vi "Weighted_Cross_Moments simple.vi"(0 "AI Cluster 1":T3={"Colour"=0, "Inst type"=enum."Pitot-static tube", "Inst name"="Manometer voltage", "Symbol"="U", "Code name"="", "Extra Info"="U", "Inst Array"=enum."PWA", "Extra Titles"=[], "Extra Values"=[], "U"=0.0, "u^2"=0.0, "u^3"=0.0, "u^4"=0.0, "Skew_u"=0.0, "Kurt_u"=0.0, "Sd Error in Mean"=0.0, "% u'/U"=0.0, "X"=0.0, "Y"=0.0, "Z"=0.0, "Timescale integral Estimate"=0.0, "Sd Error in Variance"=0.0, "Calib File"=path "", "Calib Constants"=[], "Output Position"=FALSE, "Stats"=enum."None", "Av Sampling Rate"=0.0, "Av No of Samples"=0.0, "Total Meas Time (s)"=0.0, "ADAM Ch Name"="", "Max value"=0.0, "Min value"=0.0, "Req Sample Rate Hz"=0.0, "Sync Delay Time (s)"=0.0, "Ch No"=0, "Device"="", "Use Latest Calib"=FALSE, "Port"="", "Metadata Ch Names"=[], "Metadata Ch Values"=[], "Label"=""} {"Sync Delay Time (s)" format="%.4f"; "Total Meas Time (s)" format="%_5g"; "Sd Error in Variance" format="%_3g"; "Skew_u" format="%_3g"; "% u'/U" format="%_3g"; "Sd Error in Mean" format="%_3g"; "Kurt_u" format="%_3g"; "u^4" format="%_3g"; "u^3" format="%_3g"; "U" format="%_3g"; "u^2" format="%_3g"}, 1 "AI Cluster 2":T3={"Colour"=0, "Inst type"=enum."Pitot-static tube", "Inst name"="Manometer voltage", "Symbol"="U", "Code name"="", "Extra Info"="U", "Inst Array"=enum."PWA", "Extra Titles"=[], "Extra Values"=[], "U"=0.0, "u^2"=0.0, "u^3"=0.0, "u^4"=0.0, "Skew_u"=0.0, "Kurt_u"=0.0, "Sd Error in Mean"=0.0, "% u'/U"=0.0, "X"=0.0, "Y"=0.0, "Z"=0.0, "Timescale integral Estimate"=0.0, "Sd Error in Variance"=0.0, "Calib File"=path "", "Calib Constants"=[], "Output Position"=FALSE, "Stats"=enum."None", "Av Sampling Rate"=0.0, "Av No of Samples"=0.0, "Total Meas Time (s)"=0.0, "ADAM Ch Name"="", "Max value"=0.0, "Min value"=0.0, "Req Sample Rate Hz"=0.0, "Sync Delay Time (s)"=0.0, "Ch No"=0, "Device"="", "Use Latest Calib"=FALSE, "Port"="", "Metadata Ch Names"=[], "Metadata Ch Values"=[], "Label"=""} {"Sync Delay Time (s)" format="%.4f"; "Total Meas Time (s)" format="%_5g"; "Sd Error in Variance" format="%_3g"; "Skew_u" format="%_3g"; "% u'/U" format="%_3g"; "Sd Error in Mean" format="%_3g"; "Kurt_u" format="%_3g"; "u^4" format="%_3g"; "u^3" format="%_3g"; "U" format="%_3g"; "u^2" format="%_3g"}, 2 "Time Cluster 1":T1, 3 "Time Cluster 2":T1, 5 "Shift Cluster In":cluster{"Stats":dbl[]} {"Stats" format="%.2f"}, 7 "Array 2 Time (s) offset (Default 0)":dbl, 9 "interp. method":enum16{"nearest", "linear"}(ring)=enum."linear", 11 "Index1":i32, 13 "Index2":i32) -> (17 "output cluster":T2 {"Time Window (ms)" format="%.2f"; "w^2 Paired" format="%.2f"; "u^2 Paired" format="%.2f"; "u^2w^2" format="%.2f"; "u^3w" format="%.2f"; "uw^3" format="%.2f"; "uw/u'w'" format="%.2f"; "uw^2" format="%.2f"; "u^2w" format="%.2f"; "uw" format="%.2f"}, 19 "Shift Cluster Out":cluster{"Stats":dbl[]} {"Stats" format="%.2f"})   [LabVIEW 2021]
uses:
  Controls/Analysis_info_cluster.ctl
  Controls/Inst_type.ctl
  Controls/Instrument_Array.ctl
  Controls/Correlation_cluster1.ctl
  Controls/Time_Trace_Cluster.ctl
  Globals/Meas_global.vi
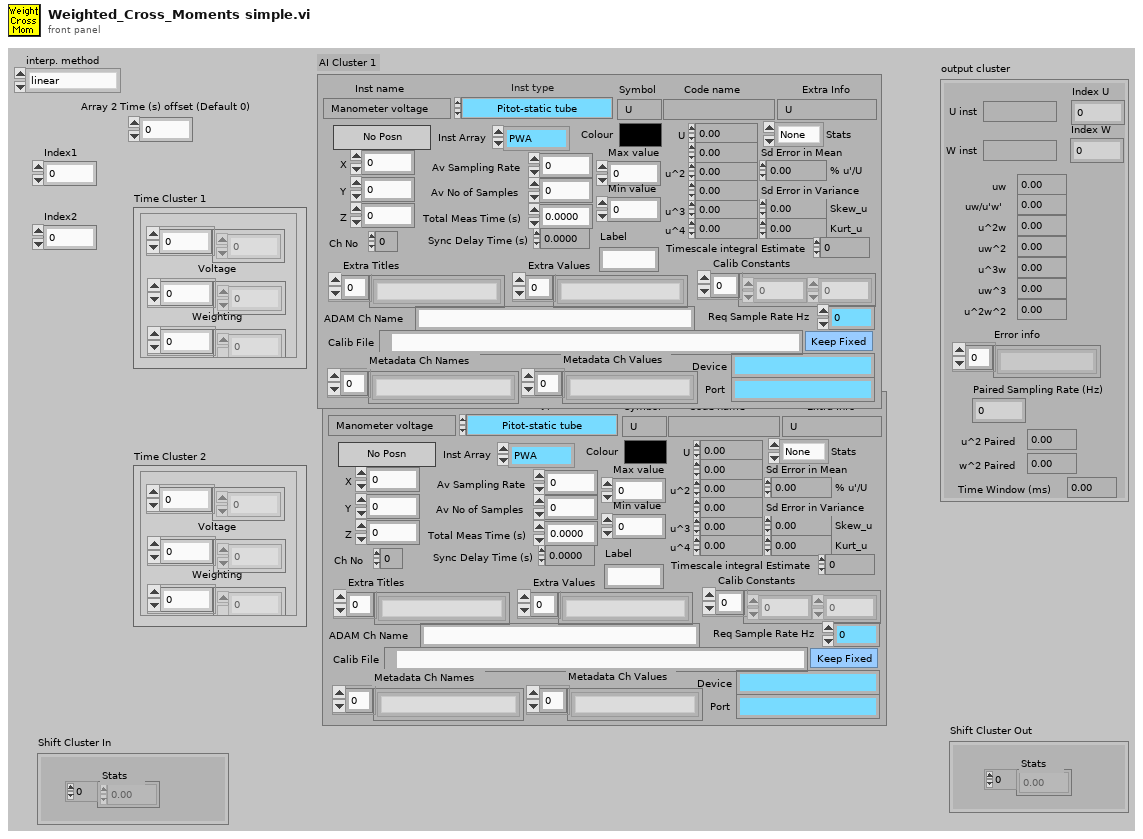
[diagram p1: front panel]
types:
  T1 = typedef "Time_Trace_Cluster.ctl" = cluster{"Weighting":dbl[], "Voltage":dbl[], "Eng Values":dbl[]}
  T2 = typedef "Correlation_cluster1.ctl" = cluster{"U inst":string, "uw":dbl, "u^2w":dbl, "uw^2":dbl, "uw/u'w'":dbl, "W inst":string, "uw^3":dbl, "u^3w":dbl, "u^2w^2":dbl, "Index U":i32, "Index W":i32, "Error info":string[], "Paired Sampling Rate (Hz)":dbl, "u^2 Paired":dbl, "w^2 Paired":dbl, "Time Window (ms)":dbl}
  T3 = typedef "Analysis_info_cluster.ctl" = cluster{"Colour":u32, "Inst type":T4, "Inst name":string, "Symbol":string, "Code name":string, "Extra Info":string, "Inst Array":T5, "Extra Titles":string[], "Extra Values":string[], "U":dbl, "u^2":dbl, "u^3":dbl, "u^4":dbl, "Skew_u":dbl, "Kurt_u":dbl, "Sd Error in Mean":dbl, "% u'/U":dbl, "X":dbl, "Y":dbl, "Z":dbl, "Timescale integral Estimate":dbl, "Sd Error in Variance":dbl, "Calib File":path, "Calib Constants":dbl[], "Output Position":bool, "Stats":enum16{"None", "Basic", "Full"}, "Av Sampling Rate":dbl, "Av No of Samples":dbl, "Total Meas Time (s)":dbl, "ADAM Ch Name":string, "Max value":dbl, "Min value":dbl, "Req Sample Rate Hz":dbl, "Sync Delay Time (s)":dbl, "Ch No":i16, "Device":string, "Use Latest Calib":bool, "Port":string, "Metadata Ch Names":string[], "Metadata Ch Values":string[], "Label":string}
  T4 = typedef "Inst_type.ctl" = enum16{"Raw voltage", "Raw with zero offsetting", "Propeller anemometer", "Pressure Transducer", "Pitot-static tube", "Hot wire", "Cross wire 1", "Cross wire 2", "Generic Linear", "Generic Polynomial", "Generic BackPoly", "Fast FID", "Thermocouple", "Cold wire", "Pulsed Wire", "LDA Vel", "LDA Tran time", "LDA Arr time", "Microphone"}
  T5 = typedef "Instrument_Array.ctl" = enum16{"PWA", "LDA", "Analogue"}
  T6 = typedef "Resample mode.ctl" = cluster{"Mode":enum16{"Index", "Interpolate"}, "Index":dbl[]}
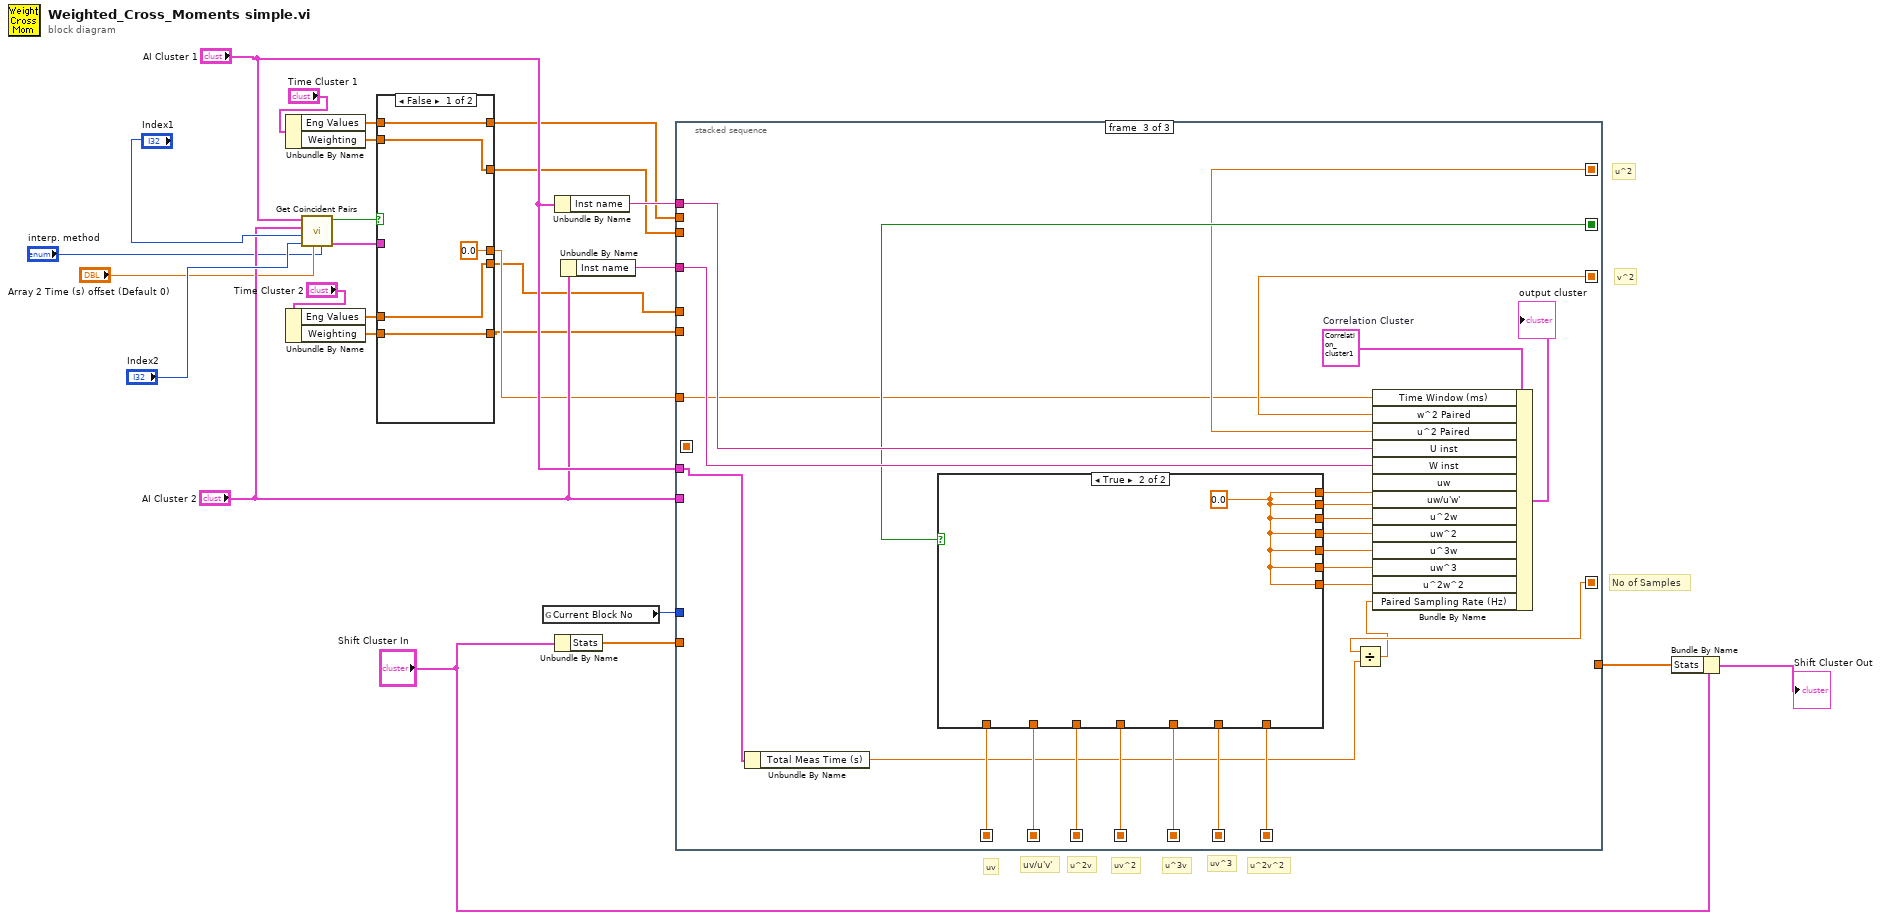
[diagram p0: block diagram]
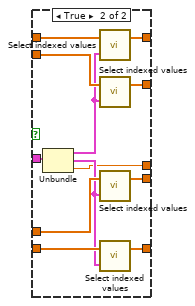
[diagram p2: hidden frame]
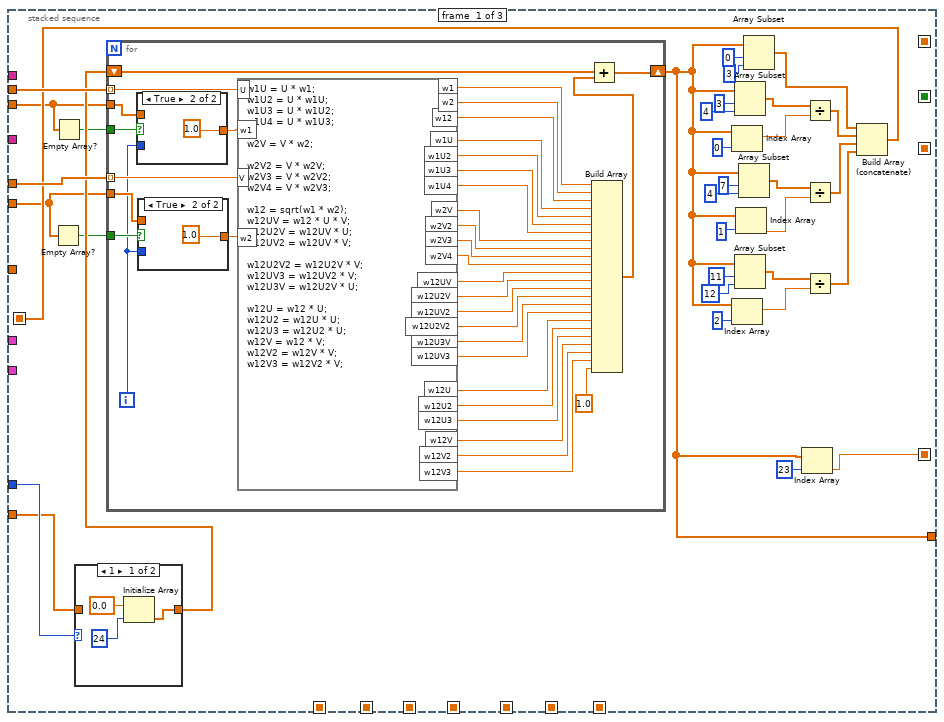
[diagram p3: hidden frame]
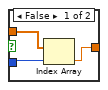
[diagram p5: hidden frame]
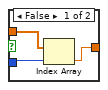
[diagram p6: hidden frame]
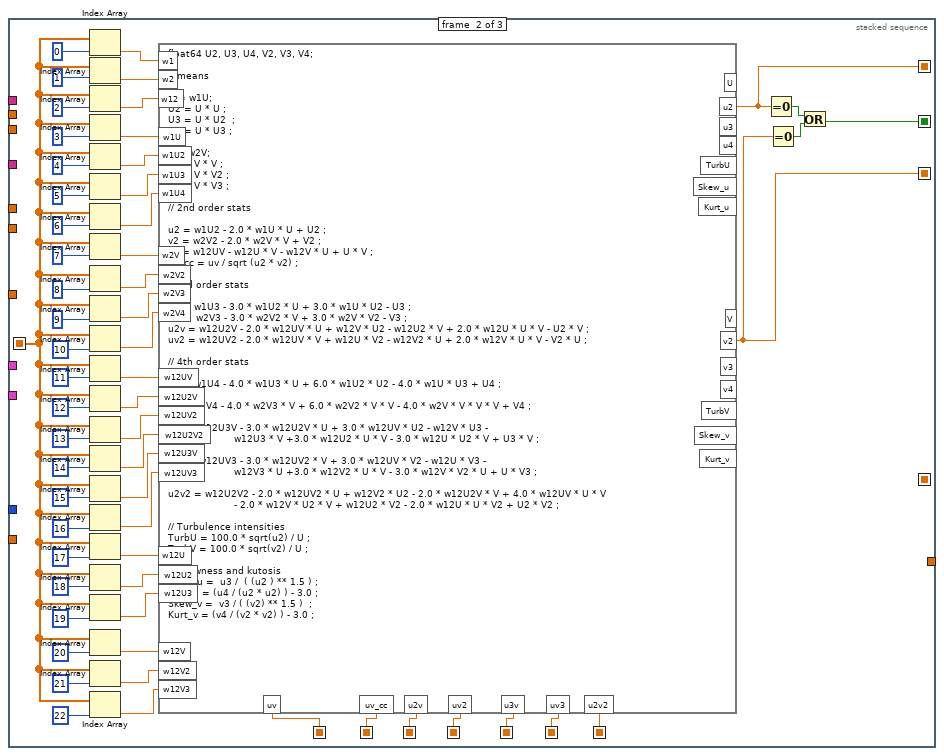
[diagram p7: hidden frame]
diagram:
  # "v^2"
  # "u^2"
  # "No of Samples"
  # "u^2v^2"
  # "uv^3"
  # "u^3v"
  # "uv^2"
  # "u^2v"
  # "uv/u'v'"
  # "uv"
  n1 = Unbundle By Name("Time Cluster 1") -> ("Eng Values"=w16:dbl[], "Weighting"=w17:dbl[])
  n2 = Unbundle By Name("Time Cluster 2") -> ("Eng Values"=w18:dbl[], "Weighting"=w19:dbl[])
  n3 = call "Get Coincident Pairs.vi"("interp. method"="interp. method", "Array 2 Time (s) offset (Default 0)"="Array 2 Time (s) offset (Default 0)", "Index2"="Index2", "Index1"="Index1", "Cluster 2"="AI Cluster 2", "Cluster 1"="AI Cluster 1") -> ("Pairs"=w14:cluster{"Cluster":T6, "Cluster":T6, dbl}, "Need to Update"=w15:bool)  [unwired: 4 in]
  n4 = case shown="False" w15 {
    tunnel: w14 -> [_ w43]
    tunnel: w16 -> [w31 w42]
    tunnel: w17 -> [w30 w41]
    tunnel: w18 -> [w29 w40]
    tunnel: w19 -> [w28 w39]
    tunnel: [w31 w35] -> w3
    tunnel: [w30 w36] -> w8
    tunnel: [w29 w37] -> w2
    tunnel: [w28 w38] -> w5
    tunnel: [0.0 w32] -> w6
    frame False {
    }
    frame True {
      n5 = Unbundle(w43) -> ("Cluster"=w33:T6, "Cluster"=w34:T6, w32:dbl)
      n6 = call "Select indexed values.vi"("Cluster"=w33, "Values"=w42) -> ("Values Out"=w35:dbl[])  [unwired: 1 in]
      n7 = call "Select indexed values.vi"("Cluster"=w33, "Values"=w41) -> ("Values Out"=w36:dbl[])  [unwired: 1 in]
      n8 = call "Select indexed values.vi"("Cluster"=w34, "Values"=w40) -> ("Values Out"=w37:dbl[])  [unwired: 1 in]
      n9 = call "Select indexed values.vi"("Cluster"=w34, "Values"=w39) -> ("Values Out"=w38:dbl[])  [unwired: 1 in]
    }
  }
  n10 = global read "Meas_global.vi" "Current Block No"() -> (w24:i32)
  n11 = Unbundle By Name("AI Cluster 1") -> ("Inst name"=w26:string)
  n12 = Unbundle By Name("Shift Cluster In") -> ("Stats"=w21:dbl[])
  n13 = Unbundle By Name("AI Cluster 2") -> ("Inst name"=w25:string)
  n14 = stacked-sequence {
    seq-local: [_ w172 _] -> [_ _ w205]
    seq-local: [_ w171 _] -> [_ _ w204]
    seq-local: [w73 _ _] -> [_ w133 _]
    seq-local: [_ w166 _] -> [_ _ w201]
    seq-local: [_ w165 _] -> [_ _ w200]
    seq-local: [_ w146 _] -> [_ _ w198]
    seq-local: [_ w145 _] -> [_ _ w196]
    seq-local: [_ w144 _] -> [_ _ w194]
    seq-local: [_ w128 _] -> [_ _ w192]
    seq-local: [w48 _ _] -> [_ _ w190]
    seq-local: [_ w127 _] -> [_ _ w187]
    seq-local: [_ w126 _] -> [_ _ w186]
    tunnel: w3 -> [w77 _ _]
    tunnel: w2 -> [w76 _ _]
    tunnel: w24 -> [w75 _ _]
    tunnel: w8 -> [w47 _ _]
    tunnel: w5 -> [w46 _ _]
    tunnel: w26 -> [_ _ w209]
    tunnel: w25 -> [_ _ w208]
    tunnel: "AI Cluster 1" -> [_ _ w191]
    tunnel: "AI Cluster 2" -> [_ _ _]
    tunnel: w21 -> [w51 _ _]
    tunnel: [w49 _ _] -> w20
    tunnel: w6 -> [_ _ w185]
    frame #0 {
      n15 = Empty Array?(array=w46) -> (empty?=w44:bool)
      n16 = Empty Array?(array=w47) -> (empty?=w45:bool)
      n17 = case shown="1" w75 {
        tunnel: [w79 w81] -> w74
        tunnel: w51 -> [_ w81]
        frame 1 {
          n18 = Initialize Array(0.0 ("Element Data"), 24 ("Dimension Size")) -> (w79:dbl[])
        }
        frame 2, Default {
        }
      }
      n19 = for {
        shift-right: [w113] -> w49
        shift-left: w74 -> [w117]
        tunnel: w47 -> [w87]
        tunnel: w77 -> [w115] mode=indexing
        tunnel: w76 -> [w114] mode=indexing
        tunnel: w46 -> [w85]
        tunnel: w45 -> [w88]
        tunnel: w44 -> [w84]
        i -> [w83]
        n20 = case shown="True" w88 {
          tunnel: [w124 1.0] -> w86
          tunnel: w83 -> [w123 _]
          tunnel: w87 -> [w122 _]
          frame False {
            n21 = Index Array(array=w122, index=w123) -> (element=w124:dbl)
          }
          frame True {
          }
        }
        n22 = case shown="True" w84 {
          tunnel: [w120 1.0] -> w82
          tunnel: w83 -> [w119 _]
          tunnel: w85 -> [w118 _]
          frame False {
            n23 = Index Array(array=w118, index=w119) -> (element=w120:dbl)
          }
          frame True {
          }
        }
        n24 = formula code="w1U = U * w1;\nw1U2 = U * w1U;\nw1U3 = U * w1U2;\nw1U4 = U * w1U3;\n\nw2V = V * w2;\n\nw2V2 = V * w2V;\nw2V3 = V * w2V2;\nw2V4 = V * w2V3;\n\nw12 = sqrt(w1 * w2);\nw12UV = w12 * U * V;\nw12U2V = w12UV * U;\nw12UV2 = w12UV * V;\n\nw12U2V2 = w12U2V * V;\nw12UV3 = w12UV2 * V;\nw12U3V = w12U2V * U;\n\nw12U = w12 * U;\nw12U2 = w12U * U;\nw12U3 = w12U2 * U;\nw12V = w12 * V;\nw12V2 = w12V * V;\nw12V3 = w12V2 * V;"("V"=w114, "U"=w115, "w1"=w86, "w2"=w82) -> ("w12UV"=w104:dbl, "w1U"=w112:dbl, "w2V"=w108:dbl, "w1U2"=w111:dbl, "w2V2"=w107:dbl, "w12U2V"=w103:dbl, "w12UV2"=w102:dbl, "w1U3"=w110:dbl, "w1U4"=w109:dbl, "w2V3"=w106:dbl, "w2V4"=w105:dbl, "w12U3V"=w100:dbl, "w12UV3"=w99:dbl, "w12U2V2"=w101:dbl, "w12U"=w95:dbl, "w12U2"=w94:dbl, "w12U3"=w93:dbl, "w12V"=w92:dbl, "w12V2"=w91:dbl, "w12V3"=w90:dbl, "w12"=w98:dbl, "w1"=w97:dbl, "w2"=w96:dbl)
        n25 = Build Array(w97, w96, w98, w112, w111, w110, w109, w108, w107, w106, w105, w104, w103, w102, w101, w100, w99, w95, w94, w93, w92, w91, w90, 1.0) -> (w116:dbl[])
        n26 = Add(x=w117, y=w116) -> (x+y=w113:dbl[])
      }
      n27 = Index Array(array=w49, index=0 ("Index")) -> (element=w69:dbl)
      n28 = Index Array(array=w49, index=2 ("Index")) -> (element=w59:dbl)
      n29 = Array Subset(array=w49, index=3 ("Array Index"), length=4) -> (w70:dbl[])
      n30 = Array Subset(array=w49, index=11 ("Array Index"), length=12) -> (w60:dbl[])
      n31 = Index Array(array=w49, index=1 ("Index")) -> (element=w66:dbl)
      n32 = Array Subset(array=w49, index=7 ("Array Index"), length=4) -> (w65:dbl[])
      n33 = Array Subset(array=w49, index=0, length=3) -> (w52:dbl[])
      n34 = Index Array(array=w49, index=23 ("Index")) -> (element=w48:dbl)
      n35 = Divide(x=w70, y=w69) -> (x/y=w57:dbl[])
      n36 = Divide(x=w65, y=w66) -> (x/y=w56:dbl[])
      n37 = Divide(x=w60, y=w59) -> (x/y=w55:dbl[])
      n38 = Build Array (concatenate)(w52, w57, w56, w55) -> (w73:dbl[])
    }
    frame #1 {
      n39 = Index Array(array=w133, index=0) -> (element=w178:dbl)
      n40 = Index Array(array=w133, index=1) -> (element=w177:dbl)
      n41 = Index Array(array=w133, index=2) -> (element=w176:dbl)
      n42 = Index Array(array=w133, index=3) -> (element=w175:dbl)
      n43 = Index Array(array=w133, index=4) -> (element=w174:dbl)
      n44 = Index Array(array=w133, index=5) -> (element=w173:dbl)
      n45 = Index Array(array=w133, index=6) -> (element=w168:dbl)
      n46 = Index Array(array=w133, index=7) -> (element=w167:dbl)
      n47 = Index Array(array=w133, index=8) -> (element=w158:dbl)
      n48 = Index Array(array=w133, index=9) -> (element=w157:dbl)
      n49 = Index Array(array=w133, index=10) -> (element=w160:dbl)
      n50 = Index Array(array=w133, index=11) -> (element=w159:dbl)
      n51 = Index Array(array=w133, index=12) -> (element=w154:dbl)
      n52 = Index Array(array=w133, index=13) -> (element=w153:dbl)
      n53 = Index Array(array=w133, index=14) -> (element=w149:dbl)
      n54 = Index Array(array=w133, index=15) -> (element=w148:dbl)
      n55 = Index Array(array=w133, index=16) -> (element=w147:dbl)
      n56 = Index Array(array=w133, index=17) -> (element=w139:dbl)
      n57 = Index Array(array=w133, index=18) -> (element=w138:dbl)
      n58 = Index Array(array=w133, index=19) -> (element=w137:dbl)
      n59 = Index Array(array=w133, index=20) -> (element=w136:dbl)
      n60 = Index Array(array=w133, index=21) -> (element=w132:dbl)
      n61 = Index Array(array=w133, index=22) -> (element=w131:dbl)
      n62 = formula code="float64 U2, U3, U4, V2, V3, V4;\n\n// means\n\nU = w1U;\nU2 = U * U ;\nU3 = U * U2  ;\nU4 = U * U3 ;\n\nV = w2V;\nV2 = V * V ;\nV3 = V * V2 ;\nV4 = V * V3 ;\n\n// 2nd order stats\n\nu2 = w1U2 - 2.0 * w1U * U + U2 ;\nv2 = w2V2 - 2.0 * w2V * V + V2 ;\nuv = w12UV - w12U * V - w12V * U + U * V ;\nuv_cc = uv / sqrt (u2 * v2) ;\n\n// 3rd order stats\n\nu3 = w1U3 - 3.0 * w1U2 * U + 3.0 * w1U * U2 - U3 ;\nv3 =  w2V3 - 3.0 * w2V2 * V + 3.0 * w2V * V2 - V3 ;\nu2v = w12U2V - 2.0 * w12UV * U + w12V * U2 - w12U2 * V + 2.0 * w12U * U * V - U2 * V ;\nuv2 = w12UV2 - 2.0 * w12UV * V + w12U * V2 - w12V2 * U + 2.0 * w12V * U * V - V2 * U ;\n\n// 4th order stats\n\nu4 = w1U4 - 4.0 * w1U3 * U + 6.0 * w1U2 * U2 - 4.0 * w1U * U3 + U4 ;\n\nv4 = w2V4 - 4.0 * w2V3 * V + 6.0 * w2V2 * V * V - 4.0 * w2V * V * V * V + V4 ;\n\nu3v = w12U3V - 3.0 * w12U2V * U + 3.0 * w12UV * U2 - w12V * U3 - \n                      w12U3 * V +3.0 * w12U2 * U * V - 3.0 * w12U * U2 * V + U3 * V ;\n\nuv3 = w12UV3 - 3.0 * w12UV2 * V + 3.0 * w12UV * V2 - w12U * V3 - \n                      w12V3 * U +3.0 * w12V2 * U * V - 3.0 * w12V * V2 * U + U * V3 ;\n\nu2v2 = w12U2V2 - 2.0 * w12UV2 * U + w12V2 * U2 - 2.0 * w12U2V * V + 4.0 * w12UV * U * V\n                      - 2.0 * w12V * U2 * V + w12U2 * V2 - 2.0 * w12U * U * V2 + U2 * V2 ; \n\n// Turbulence intensities\nTurbU = 100.0 * sqrt(u2) / U ;\nTurbV = 100.0 * sqrt(v2) / U ;\n\n// Skewness and kutosis\nSkew_u =  u3 /  ( (u2 ) ** 1.5 ) ;\nKurt_u = (u4 / (u2 * u2) ) - 3.0 ;\nSkew_v =  v3 / ( (v2) ** 1.5 )  ;\nKurt_v = (v4 / (v2 * v2) ) - 3.0 ;"("w1"=w178, "w2"=w177, "w12"=w176, "w1U2"=w174, "w1U3"=w173, "w1U"=w175, "w1U4"=w168, "w2V"=w167, "w2V2"=w158, "w2V4"=w160, "w2V3"=w157, "w12UV"=w159, "w12U2V"=w154, "w12UV2"=w153, "w12U2V2"=w149, "w12U3V"=w148, "w12UV3"=w147, "w12U2"=w138, "w12U3"=w137, "w12V"=w136, "w12V2"=w132, "w12U"=w139, "w12V3"=w131) -> ("uv"=w172:dbl, "u2"=w127:dbl, "v2"=w126:dbl, "uv_cc"=w171:dbl, "u2v"=w166:dbl, "uv2"=w165:dbl, "u3v"=w146:dbl, "uv3"=w145:dbl, "u2v2"=w144:dbl)  [unwired: 12 out]
      n63 = Equal To 0?(x=w127) -> (x = 0?=w130:bool)
      n64 = Equal To 0?(x=w126) -> (x = 0?=w129:bool)
      n65 = Or(x=w130, y=w129) -> (x .or. y?=w128:bool)
    }
    frame #2 {
      w210 = T2 {"U inst"="", "uw"=0.0, "u^2w"=0.0, "uw^2"=0.0, "uw/u'w'"=0.0, "W inst"="", "uw^3"=0.0, "u^3w"=0.0, "u^2w^2"=0.0, "Index U"=0, "Index W"=0, "Error info"=[], "Paired Sampling Rate (Hz)"=0.0, "u^2 Paired"=0.0, "w^2 Paired"=0.0, "Time Window (ms)"=0.0}  # Correlation Cluster
      n66 = Unbundle By Name(w191) -> ("Total Meas Time (s)"=w189:dbl)
      n67 = case shown="True" w192 {
        tunnel: [w217 w218] -> w206
        tunnel: w205 -> [w217 _]
        tunnel: w204 -> [w216 _]
        tunnel: [w216 w218] -> w203
        tunnel: [w215 w218] -> w202
        tunnel: w201 -> [w215 _]
        tunnel: w200 -> [w214 _]
        tunnel: [w214 w218] -> w199
        tunnel: w198 -> [w213 _]
        tunnel: [w213 w218] -> w197
        tunnel: w196 -> [w212 _]
        tunnel: [w212 w218] -> w195
        tunnel: w194 -> [w211 _]
        tunnel: [w211 w218] -> w193
        frame False {
        }
        frame True {
          w218 = 0.0 ("uv")
        }
      }
      n68 = Divide(x=w190, y=w189) -> (x/y=w188:dbl)
      n69 = Bundle By Name(cluster=w210, "Time Window (ms)"=w185, "w^2 Paired"=w186, "u^2 Paired"=w187, "U inst"=w209, "W inst"=w208, "uw"=w206, "uw/u'w'"=w203, "u^2w"=w202, "uw^2"=w199, "u^3w"=w197, "uw^3"=w195, "u^2w^2"=w193, "Paired Sampling Rate (Hz)"=w188) -> (→"output cluster":T2)
    }
  }
  n70 = Bundle By Name(cluster="Shift Cluster In", "Stats"=w20) -> (→"Shift Cluster Out":cluster{"Stats":dbl[]})
